vi "GDSArray_RemoveDuplicatesInVariantArray.vi"(1 "array":variant[](array[variant]), 5 "error in (no error)":errorcluster) -> (15 "array out":variant[](array[variant]), 19 "error out":errorcluster)   [LabVIEW 2016]
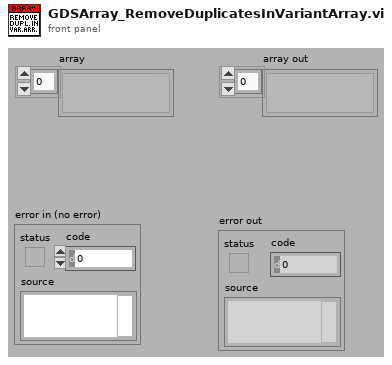
[diagram p1: front panel]
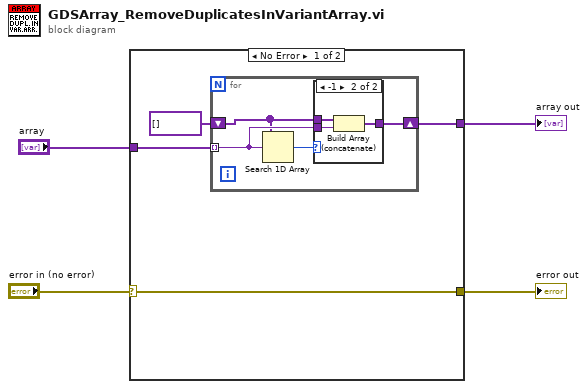
[diagram p0: block diagram]
diagram:
  n1 = case shown="No Error" "error in (no error)" {
    selector: "error in (no error)" -> [w5 w17]
    tunnel: "array" -> [w8 w18]
    tunnel: [w6 w18] -> w3
    tunnel: [w5 w17] -> w1
    frame No Error {
      n2 = for {
        tunnel: w8 -> [w10] mode=indexing
        shift-right: [w11] -> w6
        shift-left: variant[] [] -> [w9]
        n3 = Search 1D Array(1D array=w9, element=w10) -> (index of element=w12:i32)  [unwired: 1 in]
        n4 = case shown="-1" w12 {
          tunnel: [w13 w16] -> w11
          tunnel: w10 -> [_ w15]
          tunnel: w9 -> [w13 w14]
          frame Default {
          }
          frame -1 {
            n5 = Build Array (concatenate)(w14, w15) -> (w16:variant[])
          }
        }
      }
    }
    frame Error {
    }
  }
  "array out" <- w3
  "error out" <- w1
